vi "Parse Desired Parameters.vi"(7 "StringIn":string) -> (4 "Parameter1":u16, 6 "Setpoint1":dbl, 8 "Parameter2":u16, 10 "Setpoint2":dbl, 15 "Setpoint3":dbl)   [LabVIEW 2013]
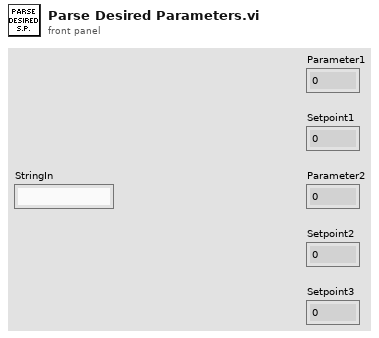
[diagram p1: front panel]
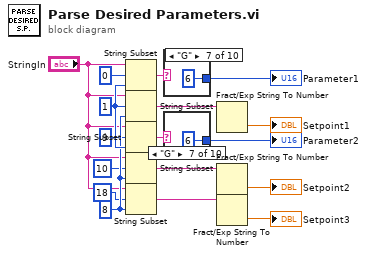
[diagram p0: block diagram]
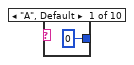
[diagram p2: hidden frame]
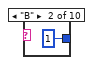
[diagram p3: hidden frame]
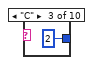
[diagram p4: hidden frame]
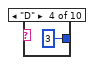
[diagram p5: hidden frame]
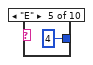
[diagram p6: hidden frame]
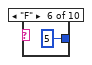
[diagram p7: hidden frame]
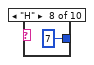
[diagram p8: hidden frame]
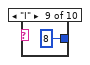
[diagram p9: hidden frame]
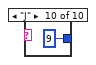
[diagram p10: hidden frame]
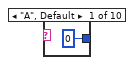
[diagram p11: hidden frame]
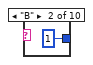
[diagram p12: hidden frame]
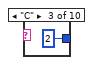
[diagram p13: hidden frame]
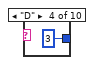
[diagram p14: hidden frame]
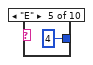
[diagram p15: hidden frame]
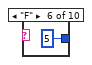
[diagram p16: hidden frame]
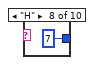
[diagram p17: hidden frame]
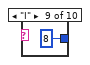
[diagram p18: hidden frame]
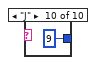
[diagram p19: hidden frame]
diagram:
  w15 = 8 ("length (rest)")
  w16 = 1 ("offset (0)")
  n1 = String Subset(string="StringIn", offset (0)=0, length (rest)=w16) -> (substring=w10:string)
  n2 = String Subset(string="StringIn", offset (0)=w16, length (rest)=w15) -> (substring=w9:string)
  n3 = String Subset(string="StringIn", offset (0)=9, length (rest)=w16) -> (substring=w11:string)
  n4 = String Subset(string="StringIn", offset (0)=10, length (rest)=w15) -> (substring=w8:string)
  n5 = String Subset(string="StringIn", offset (0)=18, length (rest)=w15) -> (substring=w7:string)
  n6 = case shown="\"G\"" w10 {
    tunnel: [u16 0 u16 1 u16 2 u16 3 u16 4 u16 5 u16 6 u16 7 u16 8 u16 9] -> w6
    frame "A", Default {
    }
    frame "B" {
    }
    frame "C" {
    }
    frame "D" {
    }
    frame "E" {
    }
    frame "F" {
    }
    frame "G" {
    }
    frame "H" {
    }
    frame "I" {
    }
    frame "J" {
    }
  }
  "Parameter1" <- w6
  n7 = case shown="\"G\"" w11 {
    tunnel: [u16 0 u16 1 u16 2 u16 3 u16 4 u16 5 u16 6 u16 7 u16 8 u16 9] -> w4
    frame "A", Default {
    }
    frame "B" {
    }
    frame "C" {
    }
    frame "D" {
    }
    frame "E" {
    }
    frame "F" {
    }
    frame "G" {
    }
    frame "H" {
    }
    frame "I" {
    }
    frame "J" {
    }
  }
  "Parameter2" <- w4
  n8 = Fract/Exp String To Number(string=w9) -> (number=→"Setpoint1":dbl)  [unwired: 3 in, 1 out]
  n9 = Fract/Exp String To Number(string=w8) -> (number=→"Setpoint2":dbl)  [unwired: 3 in, 1 out]
  n10 = Fract/Exp String To Number(string=w7) -> (number=→"Setpoint3":dbl)  [unwired: 3 in, 1 out]
